vi "ImageSource Write.vi"(4 "error in (no error)":errorcluster, 5 "Value":T2, 6 "Container State":T7, 7 "Display State In":T1={"ImageSource"=enum."Camera", "IMAQdx Cam"=refnum, "WorkDir"=path "", "Image Name Prefix"="", "ROI"={"Global Rectangle"=[], "Contours"=[]}, "BG Image"=refnum, "Display Image"=refnum, "Display settings"={"Min. Thresh."=0.0, "X"=0.0, "Y"=0.0, "ShowLineout"=FALSE, "ScaleParts"=10, "ShowLegende"=FALSE, "Target Cross"=FALSE, "Centroid Cross"=FALSE, "Target color"=16777226, "Centroid color"=16711680, "calibr. mm/px"=0.0}, "Mask image"=refnum, "ConfigDir"=path "", "Display ref"=refnum, "Saved ROIs"=[], "Selected ROI"="", "Analyze Objects"=[], "Analysis Params"=variant, "Analysis Results"=variant, "Overlays?"=[], "Ref Palette type"=refnum, "Time in Filename?"=TRUE, "Save Report?"=TRUE, "Appl Params"=variant, "Show ZoomBtn?"=TRUE, "Image file"=path ""} {"ROI"."Contours"."Type" items=["No Selection", "Point", "Line", "Rectangle", "Oval", "Polygon", "Freehand Region", "Annulus", "Unused2", "Unused3", "Broken Line", "Freehand Line", "Rotated Rectangle"]}) -> (0 "error out":errorcluster, 3 "Display State Out":T1={"ImageSource"=enum."Camera", "IMAQdx Cam"=refnum, "WorkDir"=path "", "Image Name Prefix"="", "ROI"={"Global Rectangle"=[], "Contours"=[]}, "BG Image"=refnum, "Display Image"=refnum, "Display settings"={"Min. Thresh."=0.0, "X"=0.0, "Y"=0.0, "ShowLineout"=FALSE, "ScaleParts"=10, "ShowLegende"=FALSE, "Target Cross"=FALSE, "Centroid Cross"=FALSE, "Target color"=16777226, "Centroid color"=16711680, "calibr. mm/px"=0.0}, "Mask image"=refnum, "ConfigDir"=path "", "Display ref"=refnum, "Saved ROIs"=[], "Selected ROI"="", "Analyze Objects"=[], "Analysis Params"=variant, "Analysis Results"=variant, "Overlays?"=[], "Ref Palette type"=refnum, "Time in Filename?"=TRUE, "Save Report?"=TRUE, "Appl Params"=variant, "Show ZoomBtn?"=TRUE, "Image file"=path ""} {"ROI"."Contours"."Type" items=["No Selection", "Point", "Line", "Rectangle", "Oval", "Polygon", "Freehand Region", "Annulus", "Unused2", "Unused3", "Broken Line", "Freehand Line", "Rotated Rectangle"]})   [LabVIEW 2020, in "POLARIS IMAQ Display.xctl"]
uses:
  POLARIS IMAQ Display.xctl
  <vilib>/_xctls/Container State.ctl
  ImageSource.ctl
  State.ctl
  IMAQdx Cam/IMAQdx Cam.lvclass
  <vilib>/vision/Image Controls.llb/IMAQ Image.ctl
  DisplaySettings.ctl
  Named ROI.ctl
  Analyze Classes/Analyze BaseClass/Analyze BaseClass.lvclass
  Palette.ctl
  <vilib>/_xctls/XControlSupport.lvlib
panel:
  # "Replace the Value Control below with a Control of desired type.\nDo not remove this Control or the others from the connector pane.\nDo not change the connector pane pattern.\nThe Value control should always be the third terminal from top on the input side in the connector pane."
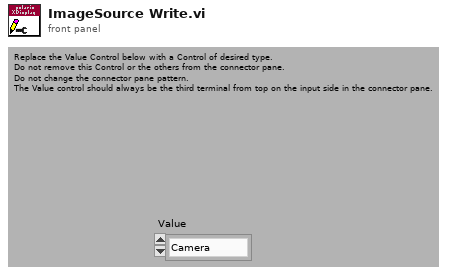
[diagram p1: front panel]
types:
  T1 = typedef "POLARIS IMAQ Display.xctl/State.ctl" = cluster{"ImageSource":T2, "IMAQdx Cam":refnum<class "IMAQdx Cam.lvclass">, "WorkDir":path, "Image Name Prefix":string, "ROI":T3, "BG Image":T4, "Display Image":T4, "Display settings":T5, "Mask image":T4, "ConfigDir":path, "Display ref":refnum<vi>, "Saved ROIs":T6[], "Selected ROI":string, "Analyze Objects":refnum<class "Analyze BaseClass.lvclass">[], "Analysis Params":variant, "Analysis Results":variant, "Overlays?":bool[], "Ref Palette type":refnum<vi>, "Time in Filename?":bool, "Save Report?":bool, "Appl Params":variant, "Show ZoomBtn?":bool, "Image file":path}
  T2 = typedef "POLARIS IMAQ Display.xctl/ImageSource.ctl" = enum16{"Camera", "File"}
  T3 = typedef "ROI Descriptor" = cluster{"Global Rectangle":i32[], "Contours":cluster{"ID":enum32{"External", "Internal"}, "Type":u32, "Coordinates":i32[]}[]}
  T4 = typedef "IMAQ Image.ctl" = refnum<image>
  T5 = typedef "POLARIS IMAQ Display.xctl/DisplaySettings.ctl" = cluster{"Min. Thresh.":sgl, "X":dbl, "Y":dbl, "ShowLineout":bool, "ScaleParts":i32, "ShowLegende":bool, "Target Cross":bool, "Centroid Cross":bool, "Target color":u32, "Centroid color":u32, "calibr. mm/px":sgl}
  T6 = typedef "POLARIS IMAQ Display.xctl/Named ROI.ctl" = cluster{"ROI":cluster{"Global Rectangle":i32[], "Contours":cluster{"Contour Type":u32, "ROI Type":u32, "Points":i32[]}[]}, "Name":string}
  T7 = typedef "XControlSupport.lvlib/Container State.ctl" = cluster{"Indicator?":bool, "Run Mode?":bool, " Refnum":refnum<vi>}
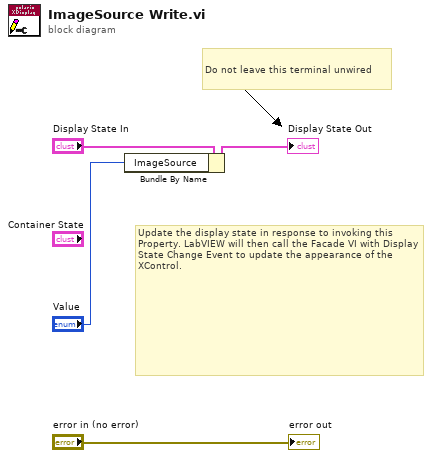
[diagram p0: block diagram]
diagram:
  # "Do not leave this terminal unwired"
  # "Update the display state in response to invoking this Property. LabVIEW will then call the Facade VI with Display State Change Event to update the appearance of the XControl."
  n1 = Bundle By Name(cluster="Display State In", "ImageSource"="Value") -> (→"Display State Out":T1)
  "error out" <- "error in (no error)"
